vi "Get Parent Item.vi"(8 "error in (no error)":errorcluster, 11 "Item Reference in":T1 format="%.0x") -> (0 "error out":errorcluster, 2 "Parent Item Reference":u64 format="%.0x", 3 "Item Reference out":T1 format="%.0x", 4 "found":bool)   [LabVIEW 2013, in "Hierarchy Framework.lvlib" / "Item.lvclass"]
doc: "Returns a reference to the parent item of the item specified by <B>Item Reference in</B>."
uses:
  Item.lvclass
  Ctls/Item Reference.ctl
  Generic/Generic.lvclass
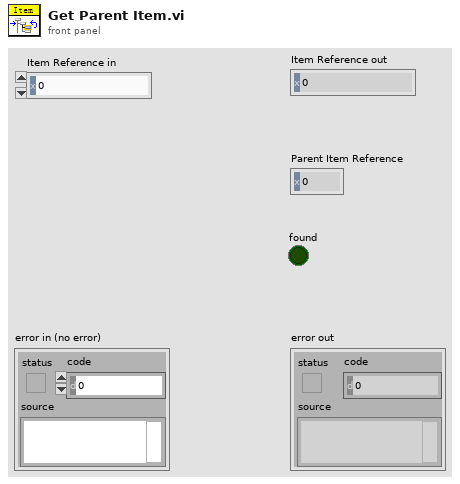
[diagram p1: front panel]
types:
  T1 = typedef "Hierarchy Framework.lvlib/Item.lvclass/Item Reference.ctl" = u64
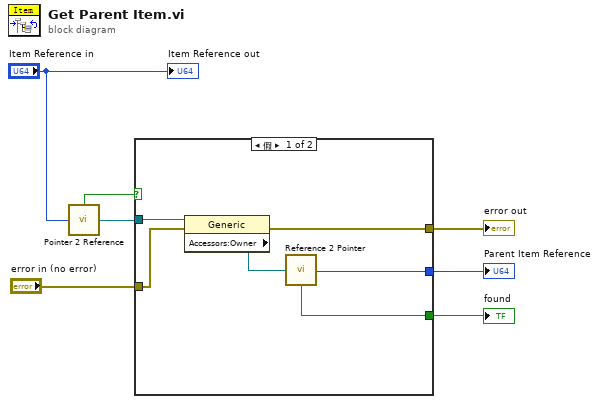
[diagram p0: block diagram]
diagram:
  n1 = call "Pointer 2 Reference.vi"("Pointer"="Item Reference in") -> ("Not A Refnum?"=w4:bool, "Generic Reference"=w3:refnum<data-value>)
  n2 = case shown="假" w4 {
    tunnel: w3 -> [w13 _]
    tunnel: "error in (no error)" -> [w12 w14]
    tunnel: [w11 w14] -> w6
    tunnel: [w10 _] -> w1
    tunnel: [w8 _] -> w2
    frame False {
      n3 = property class="Generic"(reference=w13, error in=w12) -> (error out=w11:errorcluster, "Accessors:Owner"=w9:refnum<data-value>)  [unwired: 1 out]
      n4 = call "Reference 2 Pointer.vi"("Generic Reference"=w9) -> ("Valid?"=w8:bool, "Pointer"=w10:u64)
    }
    frame True {
    }
  }
  "error out" <- w6
  "found" <- w2
  "Parent Item Reference" <- w1
  "Item Reference out" <- "Item Reference in"
